vi "Cerca celle.vi"(8 "error in (no error)":errorcluster, 11 "report in":T1) -> (0 "error out":errorcluster, 2 "Celle da riempire":string[](array[string]), 3 "report out":T1)   [LabVIEW 2022 SP3]
uses:
  <vilib>/Utility/NIReport.llb/Generate Report Object Reference.ctl
  <vilib>/Utility/NIReport.llb/NI_report.lvclass
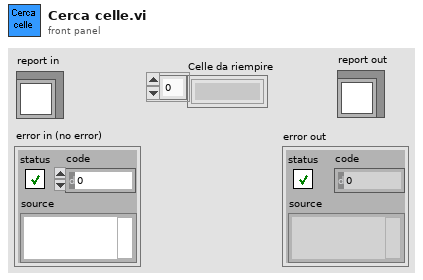
[diagram p1: front panel]
types:
  T1 = typedef "Generate Report Object Reference.ctl" = refnum<class "NI_report.lvclass">
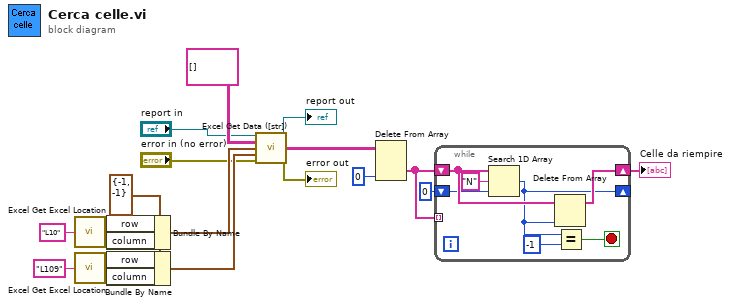
[diagram p0: block diagram]
diagram:
  w9 = cluster{"row":i32, "column":i32} {"row"=-1, "column"=-1} ("start (-1, -1)")
  n1 = call "Excel Get Excel Location.vi"("cell's name"="L10") -> ("row"=w19:i32, "column"=w18:i32)
  n2 = call "Excel Get Excel Location.vi"("cell's name"="L109") -> ("row"=w10:i32, "column"=w11:i32)
  n3 = Bundle By Name(cluster=w9, "row"=w19, "column"=w18) -> (w17:cluster{"row":i32, "column":i32})
  n4 = Bundle By Name(cluster=w9, "row"=w10, "column"=w11) -> (w8:cluster{"row":i32, "column":i32})
  n5 = call "Excel Get Data ([str]).vi"("report in"="report in", "data type"=string[][] [], "start (-1, -1)"=w17, "end (-1, -1)"=w8, "error in (no error)"="error in (no error)") -> ("report out"=→"report out":T1, "data"=w7:string[][], "error out"=→"error out":errorcluster)  [unwired: 8 in]
  n6 = Delete From Array(array=w7, index (col)=0 ("index (row)")) -> (deleted portion=w5:string[])  [unwired: 2 in, 1 out]
  n7 = while {
    tunnel: w5 -> [_] mode=indexing
    shift-right: [w21] -> _
    shift-left: 0 ("index of element") -> [w24]
    shift-right: [w23] -> w3
    shift-left: w5 -> [w25]
    stop <- w20 stop-if-true
    n8 = Search 1D Array(1D array=w25, element="N", start index (0)=w24) -> (index of element=w21:i32)
    n9 = Delete From Array(array=w25, index=w21) -> (array with subset deleted=w23:string[])  [unwired: 1 in, 1 out]
    n10 = Equal?(x=w21, y=i16 -1) -> (x = y?=w20:bool)
  }
  "Celle da riempire" <- w3
